vi "Rx Int Create Event.vi"(10 "phEvt":u32, 11 "devId":i32) -> (1 "devId out":i32, 2 "phEvt out":u32, 3 "function return":i32)   [LabVIEW 2013, in "CHR34XXX.lvlib"]
doc: "DLL BOOL __stdcall CHR34XXX_RxInt_Enable(IN int devId,IN BYTE Channel,IN BOOL Enabled); DLL BOOL __stdcall CHR34XXX_Asyn_RxCh_IntDepth(IN int devId,IN BYTE Channel,IN DWORD Depth); DLL BOOL __stdcall CHR34XXX_RxInt_CreateEvent(IN int devId,OUT HANDLE *phEvt);"
uses:
  CHR34XXX.lvlib
  CHR34XXX.dll
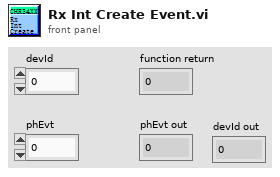
[diagram p1: front panel]
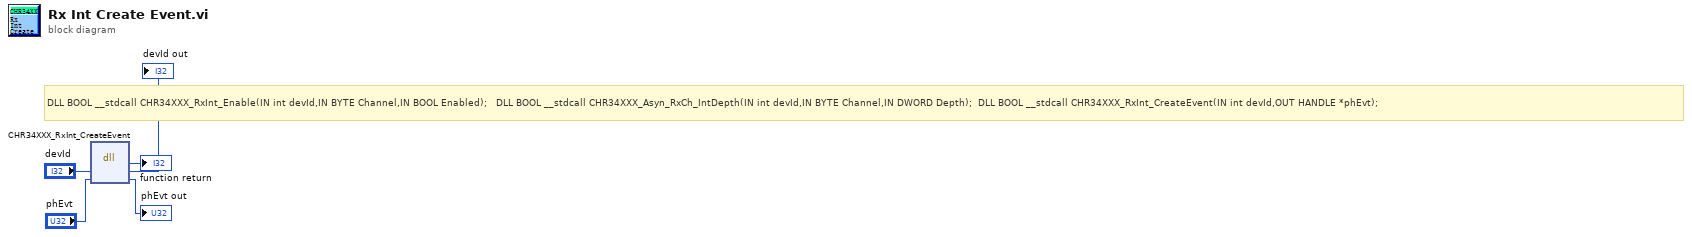
[diagram p0: block diagram]
diagram:
  # "DLL BOOL __stdcall CHR34XXX_RxInt_Enable(IN int devId,IN BYTE Channel,IN BOOL Enabled);   DLL BOOL __stdcall CHR34XXX_Asyn_RxCh_IntDepth(IN int devId,IN BYTE Channel,IN DWORD Depth);  DLL BOOL __stdcall CHR34XXX_RxInt_CreateEvent(IN int devId,OUT HANDLE *phEvt);"
  n1 = dll-call lib="C:/Users/Administrator/Desktop/CHR34XXX_lv/lv_lib/CHR34XXX.*" fn="CHR34XXX_RxInt_CreateEvent"("devId"="devId", "phEvt"="phEvt") -> (→"function return":i32, "devId"=→"devId out":i32, "phEvt"=→"phEvt out":u32)  [unwired: 3 in, 2 out]
